vi "Alias to Q.vi"(10 "Msg Q DVR Alias":string, 11 "Self Actor in":refnum<class "Self Actor.lvclass">) -> (0 "error out":errorcluster, 2 "Nested Msg Q DVR":refnum<data-value>)   [LabVIEW 2021, in "jettl.lvlib" / "Self Actor.lvclass"]
uses:
  Self Actor.lvclass
  Msg Strategy/Msg Strategy.lvclass
  Self Actor.lvclass/Self Actor.ctl
  jettl.lvlib
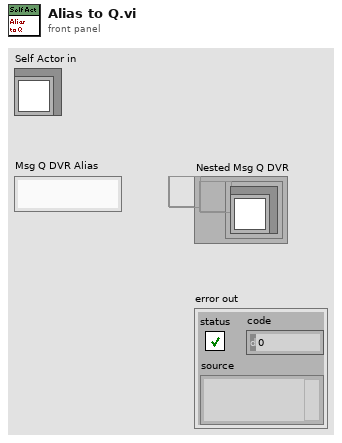
[diagram p1: front panel]
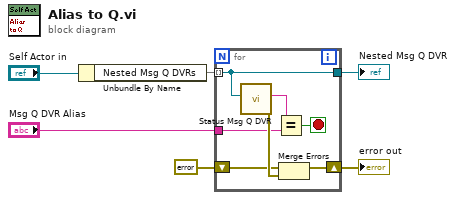
[diagram p0: block diagram]
diagram:
  n1 = Unbundle By Name("Self Actor in") -> ("Nested Msg Q DVRs"=w5:set{refnum<data-value>})
  n2 = for {
    tunnel: w5 -> [w13] mode=indexing
    tunnel: [w13] -> w3
    tunnel: "Msg Q DVR Alias" -> [w7]
    shift-right: [w8] -> w2
    shift-left: errorcluster {"status"=FALSE, "code"=0, "source"=""} ("error IO") -> [w9]
    stop <- w10 stop-if-true
    n3 = call "Status Msg Q DVR.vi"("Msg Q DVR"=w13) -> ("error out"=w11:errorcluster, "Msg Q DVR Alias"=w12:string)  [unwired: 9 in]
    n4 = Equal?(x=w12, y=w7) -> (x = y?=w10:bool)
    n5 = Merge Errors(w9, w11) -> (w8:errorcluster)
  }
  "error out" <- w2
  "Nested Msg Q DVR" <- w3
